vi "getCurrentTime.vi"(8 "error in (no error)":errorcluster, 11 "MiddlewareSALThisComponent in":refnum<class "MiddlewareSALThisComponent.lvclass">) -> (0 "error out":errorcluster, 2 "timestamp":dbl, 3 "MiddlewareSALThisComponent out":refnum<class "MiddlewareSALThisComponent.lvclass">)   [LabVIEW 2016, in "MiddlewareSALThisComponent.lvclass"]
uses:
  MiddlewareSALThisComponent.lvclass
  ts_sallv_sedspectrometer/SALLV_sedSpectrometer.lvlib
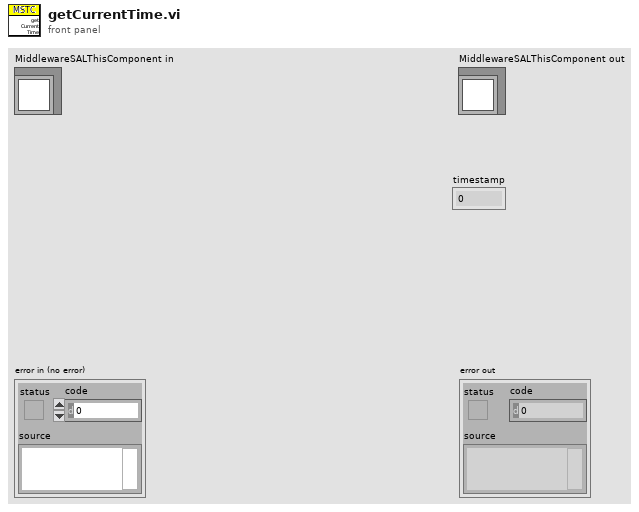
[diagram p1: front panel]
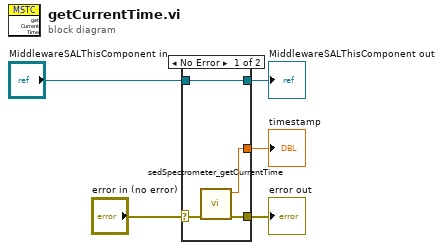
[diagram p0: block diagram]
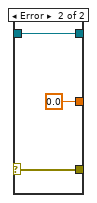
[diagram p2: hidden frame]
diagram:
  n1 = case shown="No Error" "error in (no error)" {
    selector: "error in (no error)" -> [w7 w12]
    tunnel: [w6 w12] -> w4
    tunnel: [w9 w11] -> w2
    tunnel: "MiddlewareSALThisComponent in" -> [w9 w11]
    tunnel: [w8 0.0 ("timestamp")] -> w1
    frame No Error {
      n2 = call "sedSpectrometer_getCurrentTime.vi"("error in (no error)"=w7) -> ("error out"=w6:errorcluster, "function return"=w8:dbl)  [unwired: 9 in]
    }
    frame Error {
    }
  }
  "error out" <- w4
  "MiddlewareSALThisComponent out" <- w2
  "timestamp" <- w1
